vi "버퍼쓰기와읽기.vi"() -> ()   [LabVIEW 2018]
uses:
  variablesOFcontrol.vi
  global_var/Estop.vi
  <vilib>/Instr/_visa.llb/VISA Configure Serial Port (Instr).vi
panel:
  out "Estop?":bool
  out "숫자":i16
  out "(hi.lo)":i64=-193
  out "Upper to PCU":string
  in  "VISA resource name 2":refnum<visa-resource-name>="PCU"
  out "message":string="에러 없음" caption="메시지"
  out "PCU to Upper":string
  out "엔코더부터 끝까지 문자열":string="?ÿÿÿ"
  out "Gear(FB)":u8=2
  out "Speed0(FB)":u8
  out "Speed1(FB)":u8
  out "Steer0(FB)":u8=5
  out "Steer1(FB)":u8=1
  out "Brake(FB)":u8=1
  out "부호없는 바이트 배열":u8[](array[numeric])=[2, 0, 0, 5, 1, 1, 63, 255, 255, 255]
  out "잘라낸 STX":string="STX"
  out "잘라낸 EXT0과 1":string="\r\n"
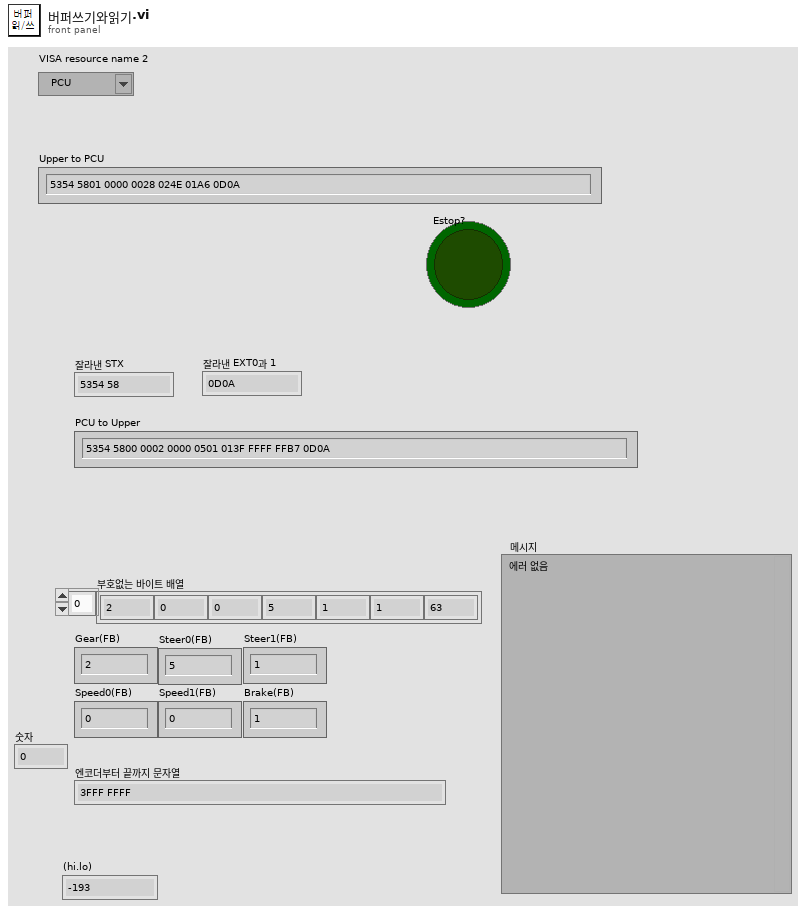
[diagram p1: front panel]
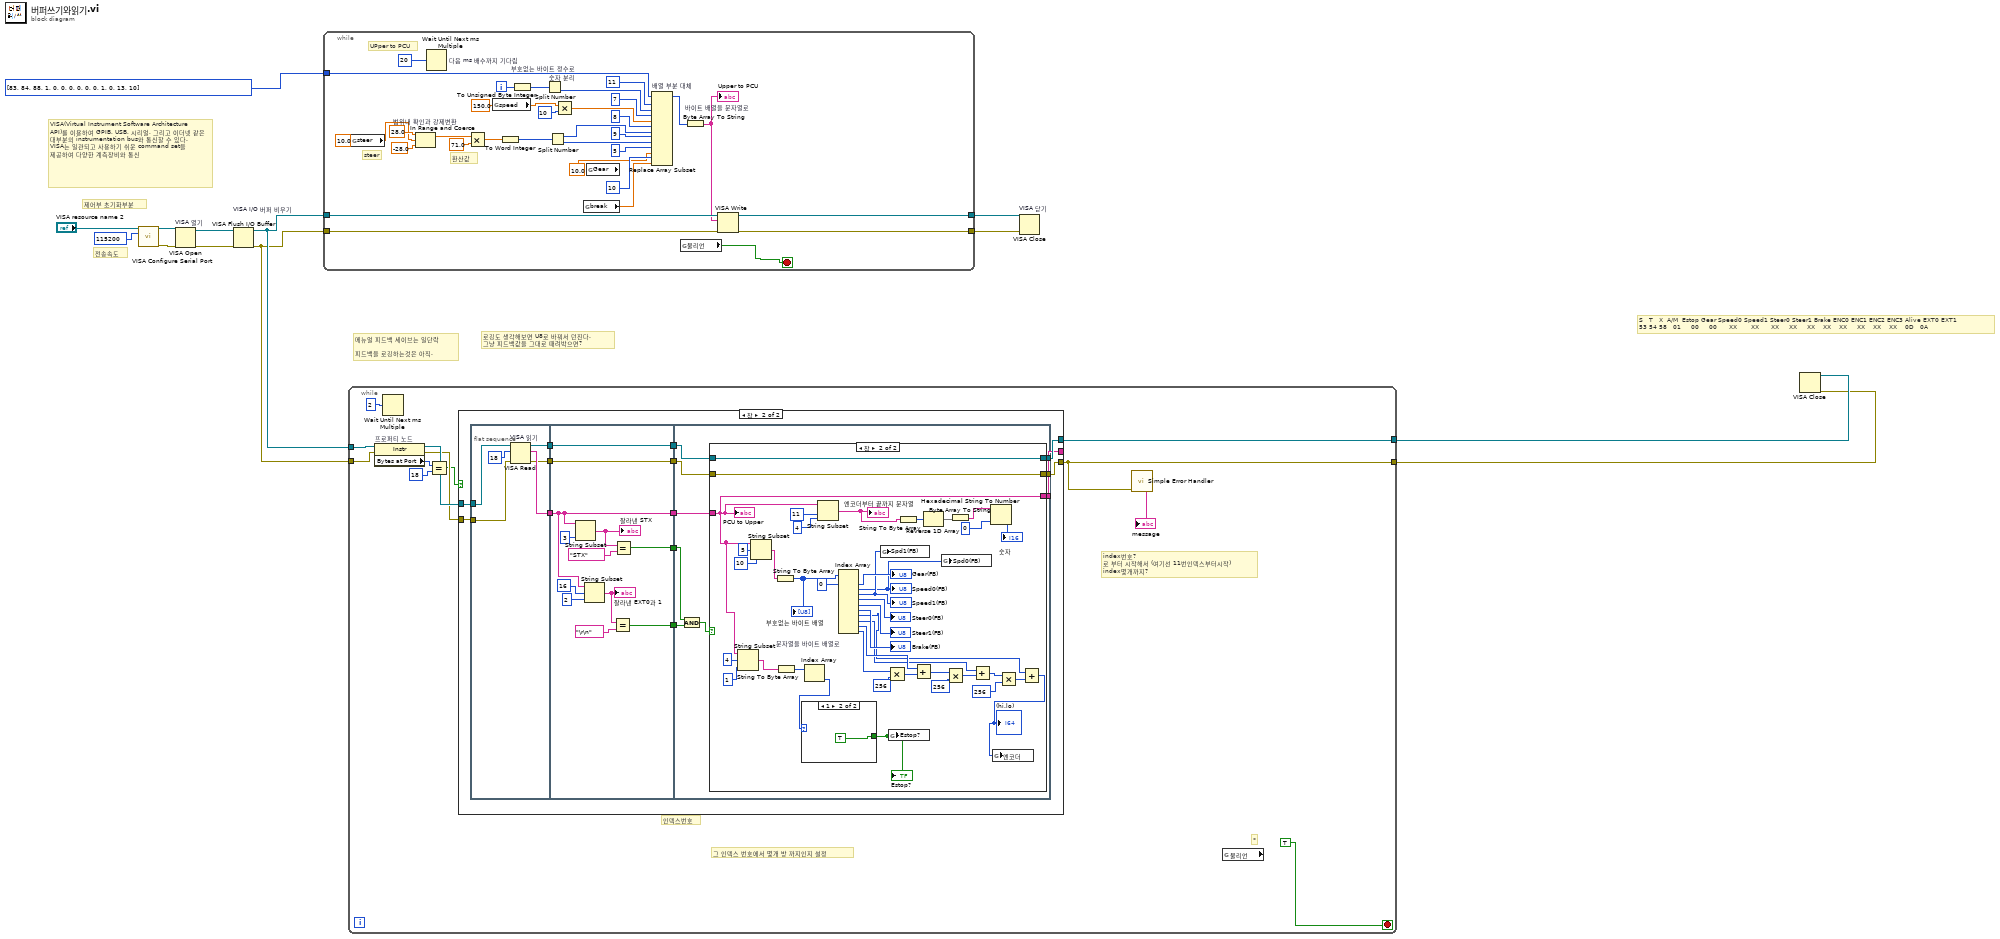
[diagram p0: block diagram]
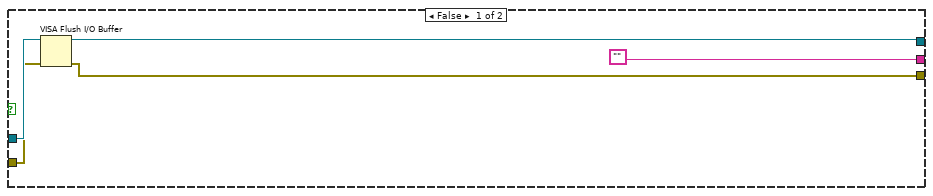
[diagram p2: hidden frame]
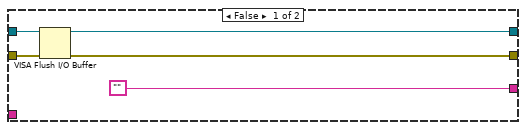
[diagram p3: hidden frame]
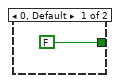
[diagram p4: hidden frame]
diagram:
  # "전송속도"
  # "VISA(Virtual Instrument Software Architecture API)를 이용하여 GPIB, USB, 시리얼, 그리고 이더넷 같은 대부분의 instrumentation bus와 통신할 수 있다. VISA는 일관되고 사용하기 쉬운 command set을 제공하여 다양한 계측장비와 통신"
  # "제어부 초기화부분"
  # "로깅도 생각해보면 U8로 바꿔서 던진다.\n그냥 피드백값을 그대로 때려박으면?"
  # "메뉴얼 피드백 세이브는 일단락\n\n피드백을 로깅하는것은 아직."
  # "S   T   X  A/M  Estop Gear Speed0 Speed1 Steer0 Steer1 Brake ENC0 ENC1 ENC2 ENC3 Alive EXT0 EXT1\n53 54 58   01     00     00      XX       XX      XX     XX     XX    XX    XX     XX    XX    XX    0D   0A"
  n1 = call-poly "VISA Configure Serial Port"("VISA resource name"="VISA resource name 2", "baud rate (9600)"=u32 115200) -> ("VISA resource name out"=w5:refnum<visa-resource-name>, "error out"=w6:errorcluster)  [unwired: 12 in]
  n2 = VISA Open "VISA 열기"(error in (no error)=w6, VISA resource name=w5) -> (VISA resource name=w4:refnum<visa-resource-name>, error out=w3:errorcluster)  [unwired: 3 in]
  n3 = VISA Flush I/O Buffer "VISA I/O 버퍼 비우기"(VISA resource name=w4, error in (no error)=w3) -> (VISA resource name out=w2:refnum<visa-resource-name>, error out=w1:errorcluster)  [unwired: 1 in]
  n4 = while {
    tunnel: w2 -> [w45]
    tunnel: w1 -> [w26]
    tunnel: [w44] -> w7
    tunnel: [w43] -> w8
    tunnel: u8[] [83, 84, 88, 1, 0, 0, 0, 0, 0, 0, 1, 0, 13, 10] ("기본값") -> [w41]
    i -> [w39]
    stop <- w17 stop-if-true
    # "steer"
    # "환산값"
    # "UPper to PCU"
    n5 = global read "variablesOFcontrol.vi" "steer"() -> ()  [unwired: 1 out]
    n6 = In Range and Coerce "범위내 확인과 강제변환"(upper limit=28.0 ("상위 리미트"), x=10.0, lower limit=-28.0 ("하위 리미트")) -> (coerced(x)=w21:dbl)  [unwired: 1 out]
    n7 = Wait Until Next ms Multiple "다음 ms 배수까지 기다림"(millisecond multiple=u32 20) -> ()  [unwired: 1 out]
    n8 = Multiply(x=w21, y=71.0) -> (x*y=w23:dbl)
    n9 = global read "variablesOFcontrol.vi" "speed"() -> ()  [unwired: 1 out]
    n10 = To Word Integer(number=w23) -> (16bit integer=w22:i16)
    n11 = To Unsigned Byte Integer "부호없는 바이트 정수로"(number=w39) -> (unsigned 8bit integer=w37:u8)
    n12 = Split Number "숫자 분리"(x=w37) -> (lo(x)=w36:u8)  [unwired: 1 out]
    n13 = Split Number(x=w22) -> (hi(x)=w29:u8, lo(x)=w28:u8)
    n14 = Multiply(x=150.0, y=u8 10) -> (x*y=w33:dbl)
    n15 = global read "variablesOFcontrol.vi" "break"() -> (w18:dbl)
    n16 = global read "variablesOFcontrol.vi" "Gear"() -> ()  [unwired: 1 out]
    n17 = Replace Array Subset "배열 부분 대체"(array=w41, new element #1=w36, index #1=11 ("인덱스"), new element #2=w33, index #2=7 ("인덱스"), new element #3=w29, index #3=8 ("인덱스"), new element #4=w28, index #4=9 ("인덱스"), new element #5=10.0, index #5=5 ("인덱스"), new element #6=w18, index #6=10 ("인덱스")) -> (w40:u8[])
    n18 = global read "프로그램종료.vi" "불리언"() -> (w17:bool)
    n19 = Byte Array To String "바이트 배열을 문자열로"(unsigned byte array=w40) -> (string=w27:string)
    "Upper to PCU" <- w27
    n20 = VISA Write(VISA resource name=w45, write buffer=w27, error in (no error)=w26) -> (VISA resource name out=w44:refnum<visa-resource-name>, error out=w43:errorcluster)  [unwired: 1 out]
  }
  n21 = while {
    tunnel: w2 -> [w56]
    tunnel: w1 -> [w52]
    tunnel: [w48] -> w13
    tunnel: [w47] -> w12
    stop <- TRUE stop-if-true
    # "*"
    # "인덱스번호"
    # "그 인덱스 번호에서 몇개 방 까지인지 설정"
    # "index번호?\n로 부터 시작해서 (여기선 11번인덱스부터시작)\nindex몇개까지?"
    n22 = property on="프로퍼티 노드" class="Instr"(reference=w56, error in=w52) -> (reference out=w55:refnum<visa-resource-name>, error out=w54:errorcluster, "Bytes at Port"=w51:u32)
    n23 = Wait Until Next ms Multiple(millisecond multiple=u32 2) -> ()  [unwired: 1 out]
    n24 = Equal?(x=w51, y=u32 18) -> (x = y?=w49:bool)
    n25 = case shown="참" w49 {
      tunnel: w55 -> [w61 w75]
      tunnel: w54 -> [w60 w74]
      tunnel: ["" w63] -> _
      tunnel: [w59 w64] -> w47
      tunnel: [w58 w65] -> w48
      frame False {
        n26 = VISA Flush I/O Buffer(VISA resource name=w61, error in (no error)=w60) -> (VISA resource name out=w58:refnum<visa-resource-name>, error out=w59:errorcluster)  [unwired: 1 in]
      }
      frame True {
        n27 = flat-sequence {
          tunnel: w75 -> [w80]
          tunnel: w74 -> [w79]
          tunnel: [w78] -> w73
          tunnel: [w77] -> w68
          tunnel: [w76] -> w66
          tunnel: w73 -> [w84]
          tunnel: [w86] -> w72
          tunnel: [w85] -> w71
          tunnel: [w84] -> w70
          tunnel: [w83] -> w69
          tunnel: w68 -> [w83]
          tunnel: [w82] -> w67
          tunnel: w66 -> [w82]
          tunnel: w72 -> [w101]
          tunnel: w71 -> [w100]
          tunnel: w70 -> [w99]
          tunnel: w69 -> [w98]
          tunnel: w67 -> [w97]
          tunnel: [w96] -> w65
          tunnel: [w95] -> w64
          tunnel: [w94] -> w63
          frame #0 {
            n28 = VISA Read "VISA 읽기"(VISA resource name=w80, byte count=u32 18 ("바이트 카운트"), error in (no error)=w79) -> (VISA resource name out=w77:refnum<visa-resource-name>, read buffer=w78:string, error out=w76:errorcluster)  [unwired: 1 out]
          }
          frame #1 {
            n29 = String Subset(string=w84, length (rest)=3 ("길이(나머지)")) -> (substring=w92:string)  [unwired: 1 in]
            "잘라낸 STX" <- w92
            n30 = String Subset(string=w84, offset (0)=16 ("오프셋(0)"), length (rest)=2 ("길이(나머지)")) -> (substring=w90:string)
            "잘라낸 EXT0과 1" <- w90
            n31 = Equal?(x=w90, y="\r\n") -> (x = y?=w86:bool)
            n32 = Equal?(x=w92, y="STX") -> (x = y?=w85:bool)
          }
          frame #2 {
            n33 = And(x=w100, y=w101) -> (x .and. y?=w102:bool)
            n34 = case shown="참" w102 {
              tunnel: w99 -> [_ w114]
              tunnel: w98 -> [w107 w147]
              tunnel: w97 -> [w106 w148]
              tunnel: [w105 w147] -> w96
              tunnel: [w104 w148] -> w95
              tunnel: ["" w114] -> w94
              frame False {
                n35 = VISA Flush I/O Buffer(VISA resource name=w107, error in (no error)=w106) -> (VISA resource name out=w105:refnum<visa-resource-name>, error out=w104:errorcluster)  [unwired: 1 in]
              }
              frame True {
                n36 = String Subset(string=w114, offset (0)=4 ("오프셋(0)"), length (rest)=1 ("길이(나머지)")) -> (substring=w113:string)
                n37 = String Subset(string=w114, offset (0)=5 ("오프셋(0)"), length (rest)=10 ("길이(나머지)")) -> (substring=w141:string)
                n38 = String To Byte Array(string=w141) -> (unsigned byte array=w142:u8[])
                "부호없는 바이트 배열" <- w142
                n39 = String To Byte Array "문자열을 바이트 배열로"(string=w113) -> (unsigned byte array=w112:u8[])
                n40 = Index Array(array=w112) -> (element=w111:u8)  [unwired: 1 in]
                n41 = case shown="1" w111 {
                  tunnel: [FALSE TRUE] -> w110
                  frame 0, Default {
                  }
                  frame 1 {
                  }
                }
                "Estop?" <- w110
                n42 = String Subset(string=w114, offset (0)=u32 11 ("초기 스캔 위치"), length (rest)=4 ("길이(나머지)")) -> (substring=w135:string)
                "엔코더부터 끝까지 문자열" <- w135
                n43 = Index Array(array=w142, index #1=0 ("인덱스")) -> (element #1=→"Gear(FB)":u8, element #2=w108:u8, element #3=w109:u8, element #4=→"Steer0(FB)":u8, element #5=→"Steer1(FB)":u8, element #6=→"Brake(FB)":u8, element #7=w118:u8, element #8=w122:u8, element #9=w126:u8, element #10=w128:u8)  [unwired: 9 in]
                "Speed0(FB)" <- w108
                "Speed1(FB)" <- w109
                n44 = global write "엔코더카운터.vi" "Spd1(FB)"(w109) -> ()
                n45 = Multiply(x=w128, y=i16 256) -> (x*y=w127:i16)
                n46 = global write "Estop.vi" "Estop?"(w110) -> ()
                n47 = String To Byte Array(string=w135) -> (unsigned byte array=w134:u8[])
                n48 = Add(x=w126, y=w127) -> (x+y=w123:i16)
                n49 = Reverse 1D Array(array=w134) -> (reversed array=w133:u8[])
                n50 = global write "엔코더카운터.vi" "Spd0(FB)"(w108) -> ()
                n51 = Multiply(x=w123, y=i16 256) -> (x*y=w125:i16)
                n52 = Byte Array To String(unsigned byte array=w133) -> (string=w132:string)
                n53 = Add(x=w122, y=w125) -> (x+y=w119:i16)
                n54 = Hexadecimal String To Number(string=w132, default (0uL)=i16 0 ("기본(0 U32)")) -> (number=→"숫자":i16)  [unwired: 1 in, 1 out]
                n55 = Multiply(x=w119, y=i16 256) -> (x*y=w121:i16)
                n56 = Add(x=w118, y=w121) -> (x+y=w117:i16)
                "(hi.lo)" <- w117
                n57 = global write "엔코더카운터.vi" "엔코더"(w117) -> ()
                "PCU to Upper" <- w114
              }
            }
          }
        }
      }
    }
    n58 = call <vilib>:"Simple Error Handler.vi"("error in (no error)"=w47) -> ("message"=→"message":string)  [unwired: 4 in, 4 out]
    n59 = global read "프로그램종료.vi" "불리언"() -> ()  [unwired: 1 out]
  }
  n60 = VISA Close "VISA 닫기"(VISA resource name=w7, error in (no error)=w8) -> ()  [unwired: 1 out]
  n61 = VISA Close(VISA resource name=w13, error in (no error)=w12) -> ()  [unwired: 1 out]
